vi "Calpoint IDs.vi"() -> ()   [LabVIEW 2015, in "ECS-RT.lvlib"]
uses:
  ECS-RT.lvlib
panel:
  out "CalPoint IDs":i32[](array[numeric])
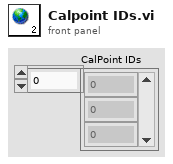
[diagram p1: front panel]
diagram:
